vi "EST.Controls.Generate.vi"(8 "error in (no error)":errorcluster, 9 "Signal":string, 10 "Input.Ref":refnum<vi>, 11 "Settings.Ref":refnum<vi>) -> (0 "error out":errorcluster)   [LabVIEW 2015, in "EST Output.lvclass"]
uses:
  EST Output.lvclass
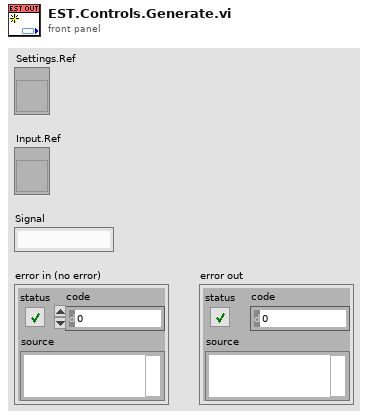
[diagram p1: front panel]
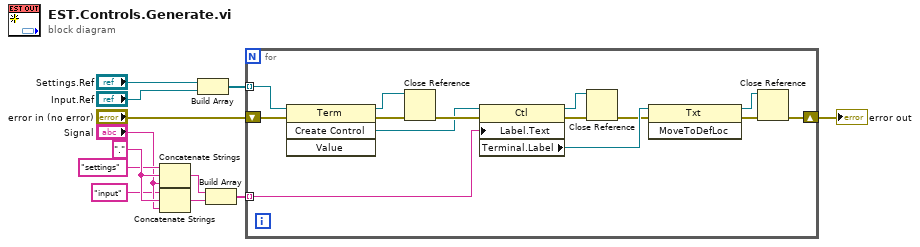
[diagram p0: block diagram]
diagram:
  w8 = "." ("string")
  n1 = Concatenate Strings("settings" ("string"), w8, "Signal") -> (w6:string)
  n2 = Concatenate Strings("input" ("string"), w8, "Signal") -> (w9:string)
  n3 = Build Array("Settings.Ref", "Input.Ref") -> (w5:refnum<vi>[])
  n4 = Build Array(w6, w9) -> (w7:string[])
  n5 = for {
    tunnel: w7 -> [w23] mode=indexing
    shift-right: [w14] -> w10
    shift-left: "error in (no error)" -> [w22]
    tunnel: w5 -> [w13] mode=indexing
    n6 = invoke class="Term" method="Create Control"(reference=w13, error in=w22) -> (reference out=w25:refnum<vi>, error out=w24:errorcluster, "Create Control"=w21:refnum<vi>)  [unwired: 2 in, 1 out]
    n7 = Close Reference(reference=w25, error in (no error)=w24) -> (error out=w26:errorcluster)
    n8 = property class="Ctl"(reference=w21, error in=w26, "Label.Text"=w23) -> (reference out=w20:refnum<vi>, error out=w18:errorcluster, "Terminal.Label"=w19:refnum<vi>)
    n9 = Close Reference(reference=w20, error in (no error)=w18) -> (error out=w17:errorcluster)
    n10 = invoke class="Txt" method="MoveToDefLoc"(reference=w19, error in=w17) -> (reference out=w15:refnum<vi>, error out=w16:errorcluster)  [unwired: 1 in, 1 out]
    n11 = Close Reference(reference=w15, error in (no error)=w16) -> (error out=w14:errorcluster)
  }
  "error out" <- w10
